vi "Obtain Control Cluster.vi"(9 "I/O":bool=TRUE, 10 "Dispense":bool=TRUE, 11 "Motion":bool=TRUE) -> (2 "Dispenser error?":bool, 3 "Control Out":T1={"I-O.lvclass"=refnum, "Gantry"=refnum, "Dispenser"="COM1"})   [LabVIEW 2021, in "Controller.lvclass"]
uses:
  Controller.lvclass
  Controllers.ctl
  I-O/I-O.lvclass
  C:/Program Files (x86)/Aerotech/A3200/LabVIEW/2010/Bin/Aerotech.A3200.dll
  Program Files (x86)/Aerotech/A3200/LabVIEW/2010/Bin/Aerotech.A3200.dll
  I-O/NI-DAQ/NI-DAQ.lvclass
  C:/Users/HEP/Documents/GitHub/Gantry/UCSB-Gantry-HEP-main/Classes/Controller/I-O/I-O.lvclass
  Drivers/Aerotech A3200/Aerotech.lvlib
  Drivers/EFD Ultimus V/EFD Ultimus V.lvlib
  Motion/A3200/A3200.lvclass
panel:
  out "error out":errorcluster
  in  "Control":T1={"I-O.lvclass"=refnum, "Gantry"=refnum, "Dispenser"="COM1"}
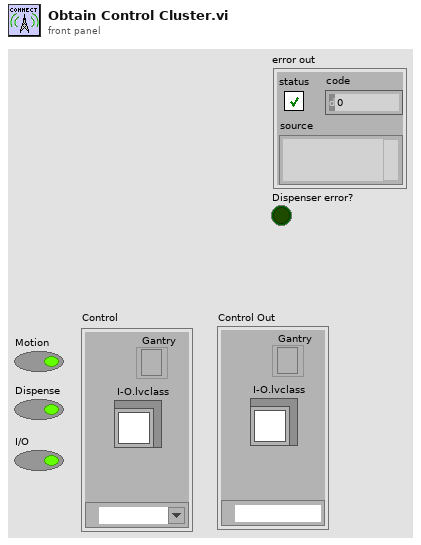
[diagram p1: front panel]
types:
  T1 = typedef "Controller.lvclass/Controllers.ctl" = cluster{"I-O.lvclass":refnum<class "I-O.lvclass">, "Gantry":refnum<k24>, "Dispenser":refnum<visa-resource-name>}
  T2 = typedef "Aerotech.lvlib/ControllerDiagPacket.ctl" = cluster{"Number of Diag Packets":i32, "Axes":T3[], "error":errorcluster}
  T3 = typedef "Aerotech.lvlib/AxisDiagPacket.ctl" = cluster{"Axis Name":string, "Analog Input 0":dbl, "Analog Input 1":dbl, "Axis Fault (num)":i32, "Axis Fault (str)":string, "Axis Fault (bits)":cluster{"AmplifierFault":bool, "AmplifierTemperatureFault":bool, "CcwEndOfTravelLimitFault":bool, "CcwSoftwareLimitFault":bool, "CommunicationLostFault":bool, "CwEndOfTravelLimitFault":bool, "CwSoftwareLimitFault":bool, "EmergencyStopFault":bool, "EncoderFault":bool, "ExternalFault":bool, "FeedbackScalingFault":bool, "GantryMisalignFault ":bool, "HallSensorFault":bool, "InPositionTimeoutFault":bool, "InternalFault":bool, "MarkerSearchFault":bool, "MaxVelocityCommandFault":bool, "MissedInterruptFault":bool, "MotorTemperatureFault":bool, "None":bool, "OverCurrentFault":bool, "PositionErrorFault":bool, "PositionFeedbackFault":bool, "PowerSupplyFault":bool, "ProbeInputFault":bool, "SafeZoneFault":bool, "VelocityErrorFault":bool, "VelocityFeedbackFault":bool, "VoltageClampFault":bool}, "Axis Status (num)":i32, "Axis Status (str)":string, "Axis Status (bits)":cluster{"BacklashActive":bool, "CalibrationEnabled1D":bool, "CalibrationEnabled2D":bool, "CommandValid":bool, "DriveAbortPending":bool, "DrivePending":bool, "Enabling":bool, "GainMappingEnabled":bool, "GantryAligned":bool, "GantryRealigning":bool, "Homed":bool, "Homing":bool, "IFOVEnabled":bool, "JogGenerating":bool, "Jogging":bool, "JoystickControl":bool, "MasterSlaveControl":bool, "MotionBlocked":bool, "MotionClamped":bool, "MoveDone":bool, "None":bool, "NotVirtual":bool, "Profiling":bool, "Stability0":bool, "Stability1":bool, "TrajectoryFiltering":bool, "WaitDone":bool}, "Current Command":sgl, "Current Error":sgl, "Current Feedback":sgl, "Digital Inputs":i32, "Digital Outputs":i32, "Drive Status":i32, "Drive Status (str)":string, "Drive Status (bits)":cluster{"AccelerationPhase":bool, "AutofocusActive":bool, "BrakeOutput":bool, "CcwEndOfTravelLimitInput":bool, "CosineEncoderError":bool, "CurrentClamp":bool, "CwEndOfTravelLimitInput":bool, "DecelerationPhase":bool, "DualLoopActive":bool, "EmergencyStopInput":bool, "Enabled":bool, "EncoderClipping":bool, "GalvoCalibrationEnabled":bool, "GalvoPowerCorrection":bool, "HallAInput":bool, "HallBInput":bool, "HallCInput":bool, "HighResolutionMode":bool, "HomeLimitInput":bool, "InPosition":bool, "InPosition2":bool, "MarkerInput":bool, "MarkerLatch":bool, "MoveActive":bool, "NoMotorSupply":bool, "None":bool, "PowerLimiting":bool, "ProgrammingFlash":bool, "ProgrammingMXH":bool, "PSOHaltLatch":bool, "ServoControl":bool, "SineEncoderError":bool}, "Position Feedback Auxiliary":dbl, "Position Command":dbl, "Position Error":dbl, "Position Feedback":dbl, "Program Position Command":dbl, "Program Position Error":dbl, "Program Position Feedback":dbl, "Velocity Command":dbl, "Velocity Error":dbl, "Velocity Feedback":dbl}
  T4 = typedef "File Paths.ctl" = cluster{"Glue Pattern Folder":path, "Carrier Tray Folder":path, "Pick Up Tool Fixture Folder":path, "Components Folder":path, "Bellows Tool Offset.txt":path, "Pick Up Tool Offset.txt":path, "Dispense Tip Offset.txt":path, "Log Files":path, "Gantry Assembly Map.txt":path, "Syringe and offset map.txt":path, "Controllers Folder":path, "Local dbase config":path}
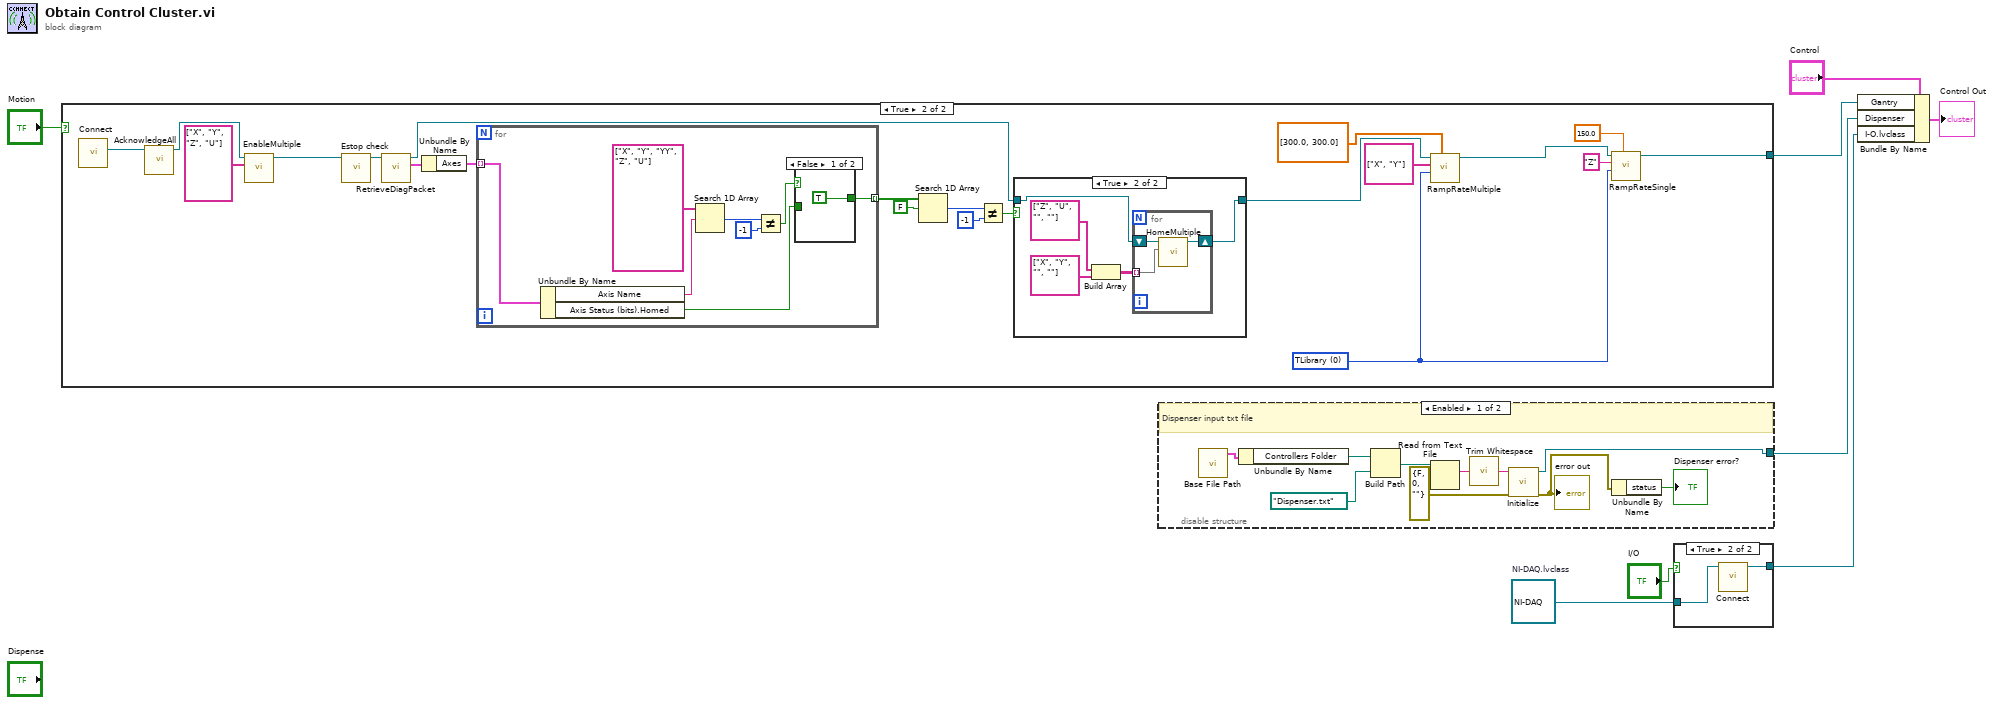
[diagram p0: block diagram]
diagram:
  w4 = refnum<class "NI-DAQ.lvclass"> refnum  # NI-DAQ.lvclass
  n1 = case shown="True" "Motion" {
    tunnel: [_ w24] -> w2
    frame False {
    }
    frame True {
      w25 = 0 items=["TLibrary", "T01", "T02", "T03", "T04", "T05", "T06", "T07", "T08", "T09", "T10", "T11", "T12", "T13", "T14", "T15", "T16", "T17", "T18", "T19", "T20", "T21", "T22", "T23", "T24", "T25", "T26", "T27", "T28", "T29", "T30", "T31"] ("task id")
      n2 = call "Connect.vi"() -> ("controller"=w10:refnum<k24>)  [unwired: 10 in, 1 out]
      n3 = call "AcknowledgeAll.vi"("controller in"=w10) -> ("controller out"=w9:refnum<k24>)  [unwired: 9 in, 1 out]
      n4 = call "EnableMultiple.vi"("axis names"=string[] ["X", "Y", "Z", "U"], "controller in"=w9) -> ("controller out"=w12:refnum<k24>)  [unwired: 8 in, 1 out]
      n5 = call "Estop check.vi"("controller in"=w12) -> ("controller out"=w15:refnum<k24>)  [unwired: 9 in, 1 out]
      n6 = call "RetrieveDiagPacket.vi"("Controller In"=w15) -> ("ControllerDiagPacket"=w14:T2, "Controller Out"=w19:refnum<k24>)  [unwired: 8 in, 1 out]
      n7 = Unbundle By Name(w14) -> ("Axes"=w13:T3[])
      n8 = for {
        tunnel: w13 -> [w37] mode=indexing
        tunnel: [w30] -> w16 mode=indexing
        n9 = Unbundle By Name(w37) -> ("Axis Name"=w35:string, "Axis Status (bits).Homed"=w31:bool)
        n10 = Search 1D Array(1D array=string[] ["X", "Y", "YY", "Z", "U"] ("axis names"), element=w35) -> (index of element=w34:i32)  [unwired: 1 in]
        n11 = Not Equal?(x=w34, y=-1) -> (x != y?=w32:bool)
        n12 = case shown="False" w32 {
          tunnel: w31 -> [_ w39]
          tunnel: [TRUE ("Homed") w39] -> w30
          frame False {
          }
          frame True {
          }
        }
      }
      n13 = Search 1D Array(1D array=w16, element=FALSE ("Homed")) -> (index of element=w20:i32)  [unwired: 1 in]
      n14 = Not Equal?(x=w20, y=-1) -> (x != y?=w21:bool)
      n15 = case shown="True" w21 {
        tunnel: w19 -> [w40 w45]
        tunnel: [w40 w44] -> w22
        frame False {
        }
        frame True {
          n16 = Build Array(string[] ["Z", "U", "", ""] ("axis names"), string[] ["X", "Y", "", ""] ("axis names")) -> (w41:string[][])
          n17 = for {
            shift-right: [w47] -> w44
            shift-left: w45 -> [w48]
            tunnel: w41 -> [w46] mode=indexing
            n18 = call "HomeMultiple.vi"("axis names"=w46, "controller in"=w48) -> ("controller out"=w47:refnum<k24>)  [unwired: 8 in, 1 out]
          }
        }
      }
      n19 = call "RampRateMultiple.vi"("ramp rates"=dbl[] [300.0, 300.0], "task id"=w25, "axis names"=string[] ["X", "Y"], "controller in"=w22) -> ("controller out"=w27:refnum<k24>)  [unwired: 6 in, 1 out]
      n20 = call "RampRateSingle.vi"("ramp rate"=150.0, "task id"=w25, "axis name"="Z", "controller in"=w27) -> ("controller out"=w24:refnum<k24>)  [unwired: 6 in, 1 out]
    }
  }
  n21 = disable-structure shown="Enabled" {
    disable-tunnel: [w58 _] -> w1
    frame Enabled {
      # "Dispenser input txt file"
      n22 = call "Base File Path.vi"() -> ("Paths Out"=w57:T4)  [unwired: 11 in]
      n23 = Unbundle By Name(w57) -> ("Controllers Folder"=w56:path)
      n24 = Build Path(base path=w56, name or relative path=path "Dispenser.txt") -> (appended path=w54:path)
      n25 = Read from Text File(file (use dialog)=w54) -> (text=w53:string)  [unwired: 3 in, 3 out]
      n26 = call <vilib>:"Trim Whitespace.vi"("string"=w53) -> ("trimmed string"=w52:string)  [unwired: 1 in]
      n27 = call "Initialize.vi"("error in (no error)"=errorcluster {"status"=FALSE, "code"=0, "source"=""}, "VISA resource name"=w52) -> ("error out"=w51:errorcluster, "VISA resource name out"=w58:refnum<visa-resource-name>)  [unwired: 8 in]
      "error out" <- w51
      n28 = Unbundle By Name(w51) -> ("status"=→"Dispenser error?":bool)
    }
    frame Disabled {
    }
  }
  n29 = case shown="True" "I/O" {
    tunnel: w4 -> [w59 w61]
    tunnel: [w59 w60] -> w6
    frame False {
    }
    frame True {
      n30 = call-dynamic "Connect.vi"("NI-DAQ in"=w61) -> ("NI-DAQ out"=w60:refnum<class "NI-DAQ.lvclass">)  [unwired: 9 in, 1 out]
    }
  }
  n31 = Bundle By Name(cluster="Control", "Gantry"=w2, "Dispenser"=w1, "I-O.lvclass"=w6) -> (→"Control Out":T1)
